vi "Config_Read_DS1102E.vi"() -> ()   [LabVIEW 2018]
panel:
  out "Waveform Data 2":waveform(dbl)(graph)
  out "M1 2":dbl
  out "M2 2":dbl
  out "M2":dbl
  out "Waveform Data":waveform(dbl)(graph)
  out "M1":dbl
  in  "Scope1":refnum<visa-resource-name>="USB0::0x1AB1::0x0488::DS1BA202100064::INSTR"
  in  "Scope2":refnum<visa-resource-name>="USB0::0x1AB1::0x0488::DS1BA202100064::INSTR"
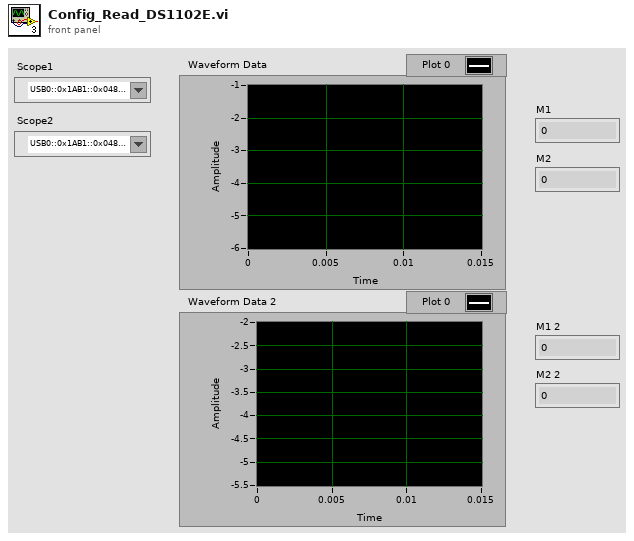
[diagram p1: front panel]
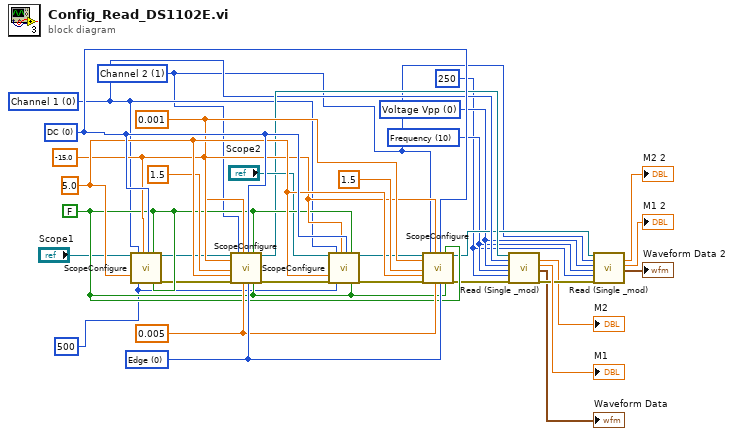
[diagram p0: block diagram]
diagram:
  w1 = u32 250 ("Timeout (10000 ms)")
  w10 = u16 0 items=["Voltage Vpp", "Voltage Max", "Voltage Min", "Amplitude", "Voltage TOP", "Voltage Base", "Voltage Average", "Voltage RMS", "Overshoot", "Preshoot", "Frequency", "Rise Time", "Fall Time", "Period", "Positive Width", "Negative Width", "Positive Duty", "Negative Duty"] ("Measurement Function (0: Voltage Vpp) 2")
  w9 = u16 10 items=["Voltage Vpp", "Voltage Max", "Voltage Min", "Amplitude", "Voltage TOP", "Voltage Base", "Voltage Average", "Voltage RMS", "Overshoot", "Preshoot", "Frequency", "Rise Time", "Fall Time", "Period", "Positive Width", "Negative Width", "Positive Duty", "Negative Duty"] ("Measurement Function (0: Voltage Vpp) 2")
  w32 = u16 0 items=["DC", "AC", "Ground"] ("Vertical Coupling (0: DC)")
  w31 = u16 0 items=["Edge", "Pulse", "Video", "Pattern", "Duration"] ("Trigger Type (0: Edge)")
  w30 = 0.005 ("offsetTime")
  w14 = u16 0 items=["Channel 1", "Channel 2", "Channel 3", "Channel 4"] ("Channel (0: Channel 1)")
  w12 = u16 1 items=["Channel 1", "Channel 2", "Channel 3", "Channel 4"] ("Channel (0: Channel 1)")
  w26 = 0.001 ("scaleTime")
  w25 = -15.0 ("offsetVoltage")
  w29 = 5.0 ("scaleVoltage")
  w16 = 500 ("Attenuation")
  w24 = FALSE
  n1 = call "ScopeConfigure.vi"("VISA resource name"="Scope1", "scaleVoltage"=w29, "Channel (0: Channel 1)"=w14, "Attenuation"=w16, "offsetVoltage"=w25, "Vertical Coupling (0: DC)"=w32, "BW Selector"=w24, "F Selector"=w24) -> ("VISA resource name out"=w23:refnum<visa-resource-name>, "error out"=w21:errorcluster)  [unwired: 10 in]
  n2 = call "ScopeConfigure.vi"("VISA resource name"=w23, "scaleTime"=w26, "triggerVoltage"=1.5, "scaleVoltage"=w29, "error in (no error)"=w21, "Channel (0: Channel 1)"=w12, "offsetVoltage"=w25, "offsetTime"=w30, "Vertical Coupling (0: DC)"=w32, "Trigger Type (0: Edge)"=w31, "BW Selector"=w24, "F Selector"=w24) -> ("VISA resource name out"=w15:refnum<visa-resource-name>, "error out"=w20:errorcluster)  [unwired: 6 in]
  n3 = call "ScopeConfigure.vi"("VISA resource name"="Scope2", "scaleVoltage"=w29, "error in (no error)"=w20, "Channel (0: Channel 1)"=w14, "Attenuation"=w16, "offsetVoltage"=w25, "Vertical Coupling (0: DC)"=w32, "BW Selector"=w24, "F Selector"=w24) -> ("VISA resource name out"=w22:refnum<visa-resource-name>, "error out"=w19:errorcluster)  [unwired: 9 in]
  n4 = call "ScopeConfigure.vi"("VISA resource name"=w22, "scaleTime"=w26, "triggerVoltage"=1.5, "scaleVoltage"=w29, "error in (no error)"=w19, "Channel (0: Channel 1)"=w12, "offsetVoltage"=w25, "offsetTime"=w30, "Vertical Coupling (0: DC)"=w32, "Trigger Type (0: Edge)"=w31, "BW Selector"=w24, "F Selector"=w24) -> ("VISA resource name out"=w13:refnum<visa-resource-name>, "error out"=w7:errorcluster)  [unwired: 6 in]
  n5 = call "Read (Single _mod).vi"("VISA resource name"=w15, "Channel (0: Channel 1)"=w14, "Measurement Function (0: Voltage Vpp) 2"=w10, "Measurement Function (0: Voltage Vpp)"=w9, "Timeout (10000 ms)"=w1, "error in (no error)"=w7) -> ("M2"=→"M2":dbl, "M1"=→"M1":dbl, "Waveform Data"=→"Waveform Data":waveform(dbl), "error out"=w8:errorcluster)  [unwired: 9 in, 1 out]
  n6 = call "Read (Single _mod).vi"("VISA resource name"=w13, "Channel (0: Channel 1)"=w12, "Measurement Function (0: Voltage Vpp) 2"=w10, "Measurement Function (0: Voltage Vpp)"=w9, "Timeout (10000 ms)"=w1, "error in (no error)"=w8) -> ("M2"=→"M2 2":dbl, "M1"=→"M1 2":dbl, "Waveform Data"=→"Waveform Data 2":waveform(dbl))  [unwired: 9 in, 2 out]
